vi "Number to String Conversion.vi"() -> ()   [LabVIEW 2020]
panel:
  in  "precision (6)":i16
  in  "width (-)":i16
  out "octal integer string":string
  out "hex integer string":string
  out "F-format string":string
  out "Engineering string":string
  out "E-format string":string
  in  "Fractional Number":dbl
  out "decimal integer string":string
  in  "Integer Number":i32
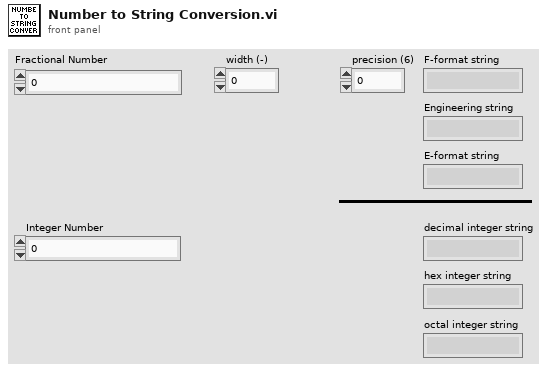
[diagram p1: front panel]
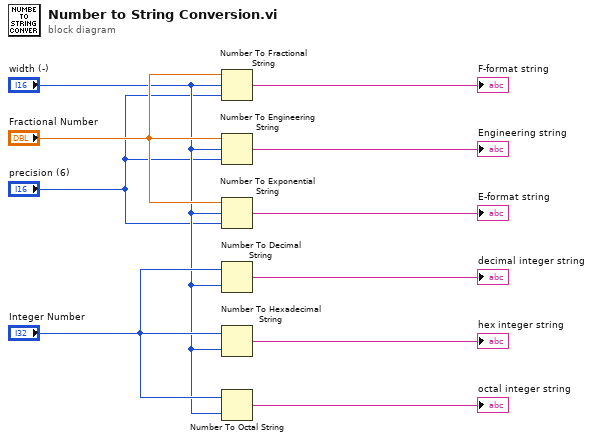
[diagram p0: block diagram]
diagram:
  n1 = Number To Fractional String(number="Fractional Number", width (-)="width (-)", precision (6)="precision (6)") -> (F-format string=→"F-format string":string)  [unwired: 1 in]
  n2 = Number To Engineering String(2:"precision (6)", 3:"width (-)", 4:"Fractional Number") -> (0:→"Engineering string":string)  [unwired: 1 in]
  n3 = Number To Exponential String(number="Fractional Number", precision (6)="precision (6)", 3:"width (-)") -> (E-format string=→"E-format string":string)  [unwired: 1 in]
  n4 = Number To Decimal String(number="Integer Number", width (-)="width (-)") -> (decimal integer string=→"decimal integer string":string)
  n5 = Number To Hexadecimal String(1:"width (-)", 2:"Integer Number") -> (0:→"hex integer string":string)
  n6 = Number To Octal String(1:"width (-)", 2:"Integer Number") -> (0:→"octal integer string":string)
